vi "test-secondcall.vi"() -> ()   [LabVIEW 2017]
panel:
  out "Array":T1(array[cluster])
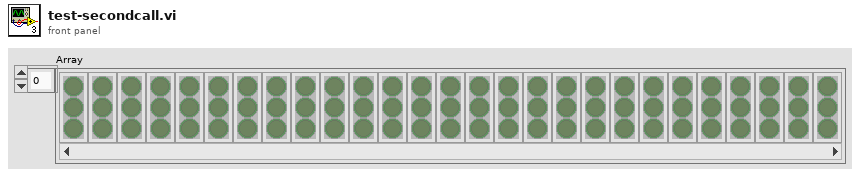
[diagram p1: front panel]
types:
  T1 = cluster{"First Call?: T/F":bool, "Second Call?: T/F":bool, "Second Call?: T/F 2":bool}[]
  T2 = cluster{"First Call?: T/F":bool, "Second Call?: T/F":bool, "Second Call?: T/F":bool}
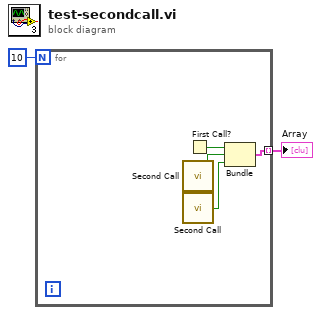
[diagram p0: block diagram]
diagram:
  n1 = for {
    N: 10 -> [_]
    tunnel: [w4] -> w1 mode=indexing
    n2 = call "Second Call.vi"() -> ("Second Call?: T/F"=w5:bool)
    n3 = call "Second Call.vi"() -> ("Second Call?: T/F"=w3:bool)
    n4 = First Call?() -> (First Call?: T/F=w6:bool)
    n5 = Bundle("First Call?: T/F"=w6, "Second Call?: T/F"=w5, "Second Call?: T/F"=w3) -> (w4:T2)  [unwired: 1 in]
  }
  "Array" <- w1
